vi "State data Look up integer key.vi"(6 "Error on not found (T)":bool=TRUE, 7 "Key [string/enum]":variant, 8 "error in (no error)":errorcluster, 10 "Value if not found (0)":i32, 11 "Fiber Auto Collimation state data in":refnum<class "Fiber Auto Collimation state data.lvclass">) -> (0 "error out":errorcluster, 1 "Integer Key found":bool, 2 "Integer Key Value":i32, 3 "Fiber Auto Collimation state data out":refnum<class "Fiber Auto Collimation state data.lvclass">)   [LabVIEW 2018, in "Fiber Auto Collimation state data.lvclass"]
doc: "Serial number of the Device Under Test."
uses:
  Fiber Auto Collimation state data.lvclass
  Fiber Auto Collimation state data.lvclass/Fiber Auto Collimation state data.ctl
  <userlib>/Recipe/Test Recipe classes/Test Recipe.lvclass
  C:/Program Files (x86)/National Instruments/LabVIEW 2018/user.lib/Recipe/nLight Recipe/nLight Recipe.lvclass
  <userlib>/Recipe/nLight Recipe/nLight Recipe.lvclass
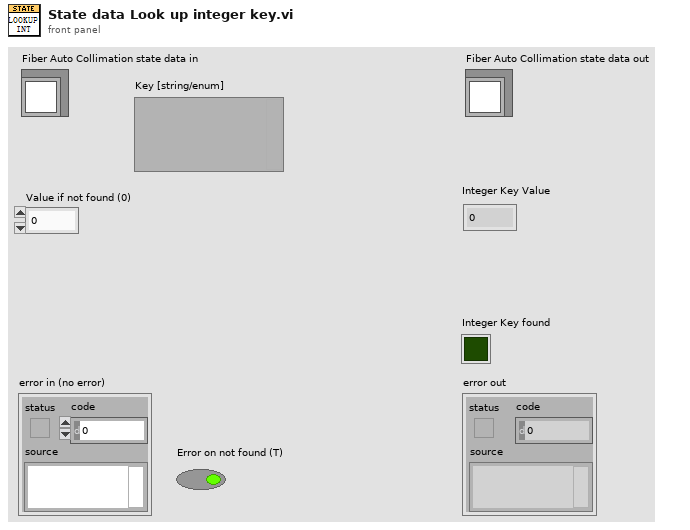
[diagram p1: front panel]
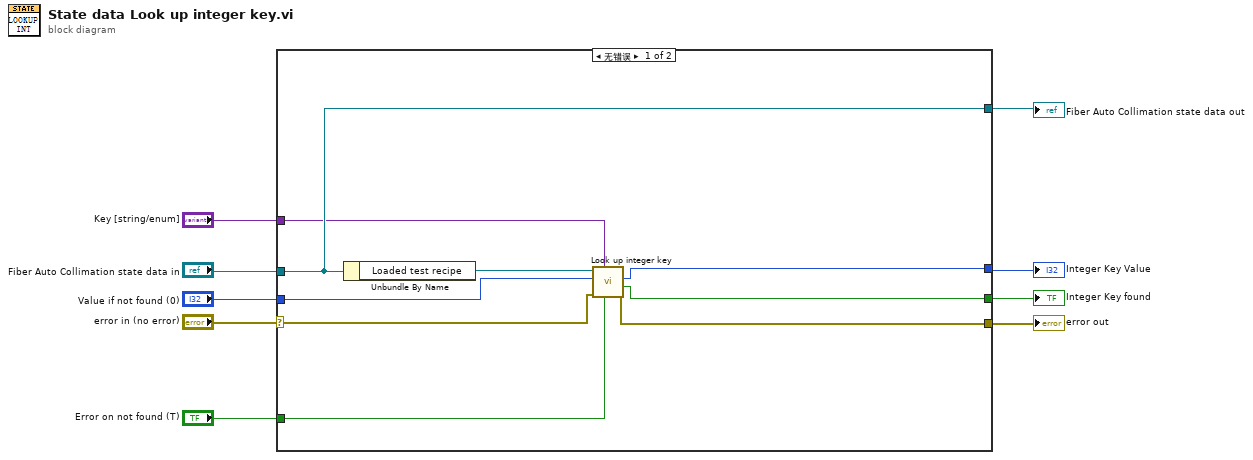
[diagram p0: block diagram]
diagram:
  n1 = case shown="无错误" "error in (no error)" {
    selector: "error in (no error)" -> [w16 w20]
    tunnel: [w11 w20] -> w8
    tunnel: [w12 w19] -> w3
    tunnel: "Fiber Auto Collimation state data in" -> [w12 w19]
    tunnel: "Key [string/enum]" -> [w10 _]
    tunnel: "Error on not found (T)" -> [w15 _]
    tunnel: [w13 _] -> w1
    tunnel: [w14 _] -> w5
    tunnel: "Value if not found (0)" -> [w17 _]
    frame No Error {
      n2 = Unbundle By Name(w12) -> ("Loaded test recipe"=w18:refnum<class "Test Recipe.lvclass">)
      n3 = call <userlib>:"Look up integer key.vi"("Error on not found (T)"=w15, "Key [string/enum]"=w10, "error in (no error)"=w16, "Value if not found (0)"=w17, "nLight Recipe in"=w18) -> ("error out"=w11:errorcluster, "Integer Key found"=w14:bool, "Integer Key Value"=w13:i32)  [unwired: 3 in, 1 out]
    }
    frame Error {
    }
  }
  "Fiber Auto Collimation state data out" <- w3
  "error out" <- w8
  "Integer Key found" <- w5
  "Integer Key Value" <- w1
